vi "Show Path.vi"(8 "error in (no error)":errorcluster, 10 "Steps":cluster{"row":i32, "col":i32}[](array[cluster]), 11 "Maze in":refnum<class "Maze.lvclass">) -> (0 "error out":errorcluster, 2 "Maze":string[][](array[string]), 3 "Maze out":refnum<class "Maze.lvclass">)   [LabVIEW 2021, in "Maze.lvclass"]
uses:
  Maze.lvclass
  Maze.lvclass/Maze.ctl
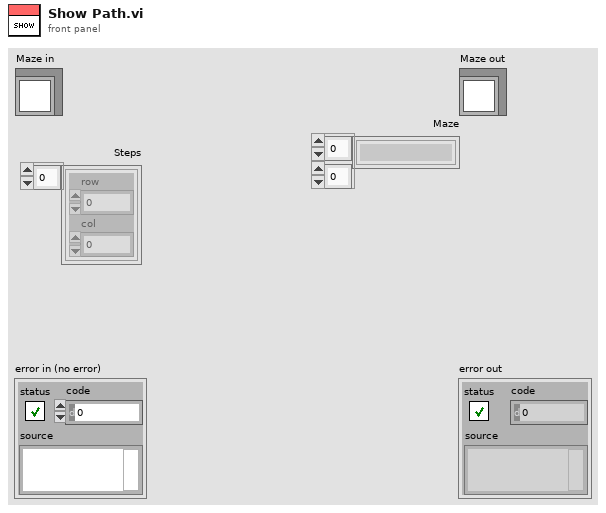
[diagram p1: front panel]
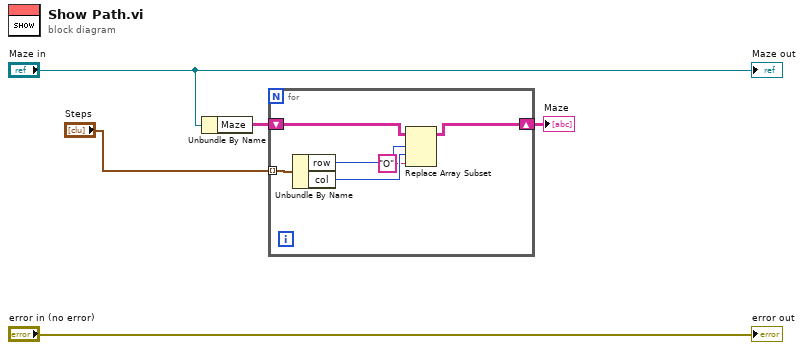
[diagram p0: block diagram]
diagram:
  n1 = Unbundle By Name("Maze in") -> ("Maze"=w3:string[][])
  n2 = for {
    tunnel: "Steps" -> [w11] mode=indexing
    shift-right: [w8] -> w2
    shift-left: w3 -> [w9]
    n3 = Unbundle By Name(w11) -> ("row"=w10:i32, "col"=w7:i32)
    n4 = Replace Array Subset(array=w9, new element="O" ("new element/subarray"), index (row)=w10, index (col)=w7) -> (w8:string[][])
  }
  "Maze" <- w2
  "error out" <- "error in (no error)"
  "Maze out" <- "Maze in"
